vi "DispenseOnly.vi"() -> ()   [LabVIEW 2019]
uses:
  Other Models/EFD Ultimus V/EFD Ultimus V.lvlib
panel:
  in  "ActualDispense":bool
  out "NewPatternPressure":dbl[](array[numeric])
  out "AmtDispensed(g)":dbl
  out "CorrectionFactor":dbl=1.0
  in  "WtFor50Psi30Sec":dbl=1.039
  in  "PaperWtWithGlue(g)":dbl
  in  "PaperWt(g)":dbl
  in  "PatternPressDefault":dbl[](array[numeric])=[30.0, 21.0, 0.0, 0.0]
  out "TimeCalculated":dbl
  out "error out":errorcluster
  in  "Serial Configuration":T1={"Baud Rate "=115200, "Parity "=0, "Data Bits "=8, "Stop Bits"=10} {"Stop Bits" items=["1.0"=10, "1.5"=15, "2.0"=20]; "Data Bits" items=["7"=7, "8"=8]; "Parity" items=["None", "Odd", "Even"]; "Baud Rate" items=["9600"=9600, "19200"=19200, "38400"=38400, "115200"=115200]}
  in  "VISA resource name":refnum<visa-resource-name>="COM5"
  in  "Time(s)":dbl=30.0
  in  "PressureSet":dbl=50.0
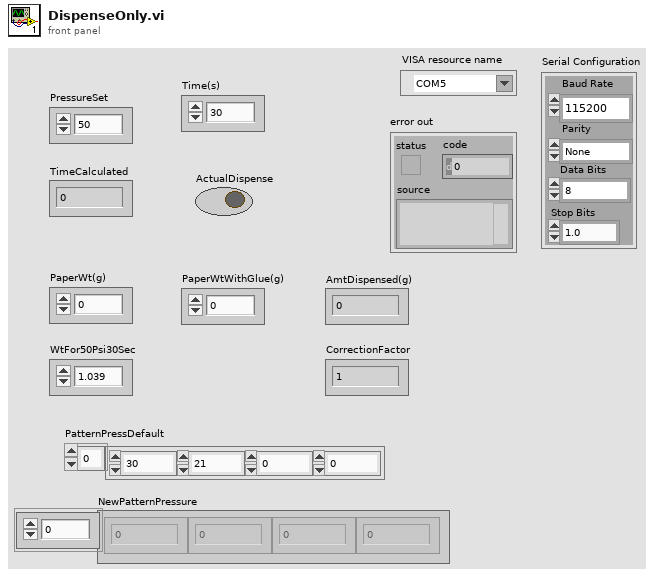
[diagram p1: front panel]
types:
  T1 = cluster{"Baud Rate ":u32, "Parity ":u16, "Data Bits ":u16, "Stop Bits":u16}
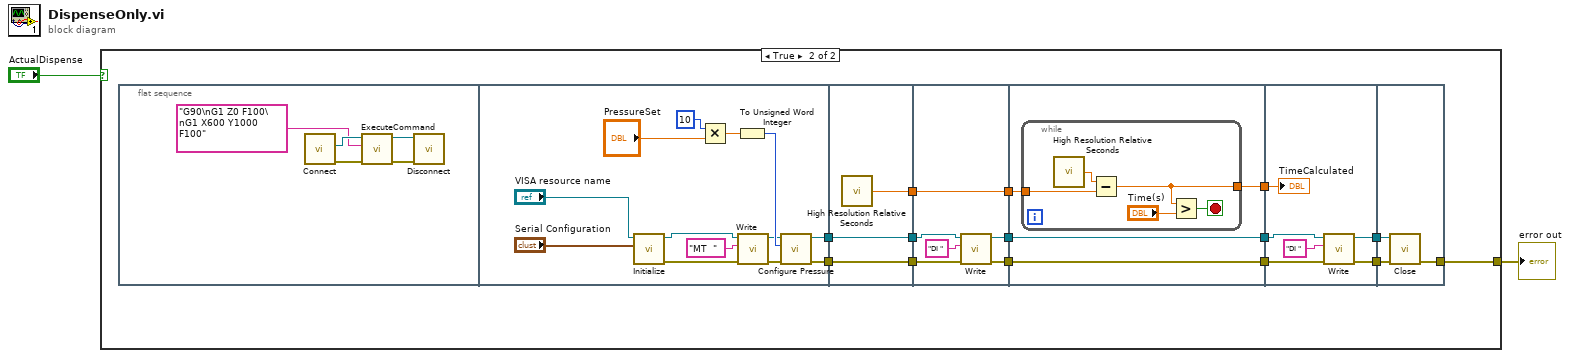
[diagram p0: block diagram]
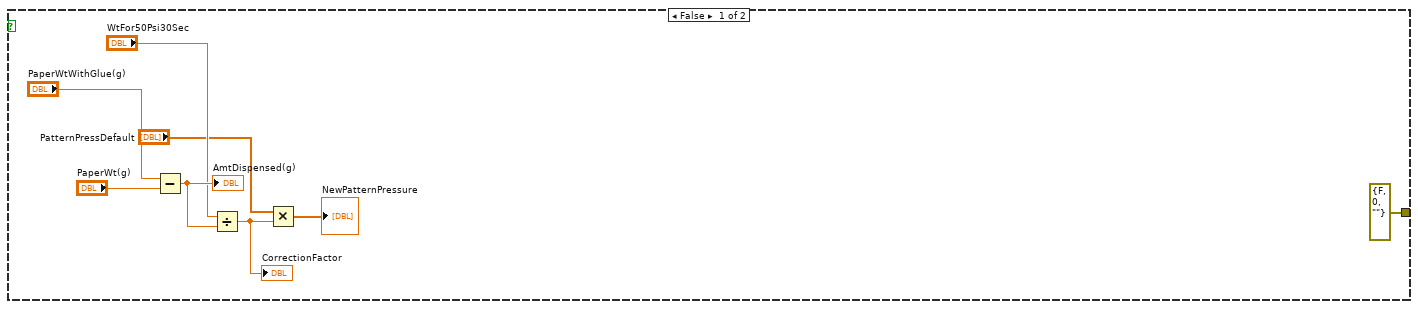
[diagram p2: hidden frame]
diagram:
  n1 = case shown="True" "ActualDispense" {
    tunnel: [errorcluster {"status"=FALSE, "code"=0, "source"=""} ("error in (no error)") w11] -> w2
    frame False {
      n2 = Subtract(x="PaperWtWithGlue(g)", y="PaperWt(g)") -> (x-y=w8:dbl)
      "AmtDispensed(g)" <- w8
      n3 = Divide(x="WtFor50Psi30Sec", y=w8) -> (x/y=w5:dbl)
      "CorrectionFactor" <- w5
      n4 = Multiply(x="PatternPressDefault", y=w5) -> (x*y=→"NewPatternPressure":dbl[])
    }
    frame True {
      n5 = flat-sequence {
        tunnel: [w30] -> w24
        tunnel: [w31] -> w23
        tunnel: [w45] -> w22
        tunnel: [w44] -> w21
        tunnel: [w43] -> w20
        tunnel: w24 -> [w45]
        tunnel: w23 -> [w44]
        tunnel: [w49] -> w19
        tunnel: [w48] -> w18
        tunnel: w22 -> [w51]
        tunnel: w21 -> [w50]
        tunnel: [w46] -> w17
        tunnel: w20 -> [w46]
        tunnel: w19 -> [w55]
        tunnel: w18 -> [w54]
        tunnel: [w55] -> w16
        tunnel: [w54] -> w15
        tunnel: w17 -> [w53]
        tunnel: [w52] -> w14
        tunnel: w16 -> [w65]
        tunnel: w15 -> [w66]
        tunnel: w14 -> [w61]
        tunnel: [w64] -> w13
        tunnel: [w63] -> w12
        tunnel: w13 -> [w69]
        tunnel: w12 -> [w68]
        tunnel: [w67] -> w11
        frame #0 {
          n6 = call "Connect.vi"() -> ("error out"=w28:errorcluster, "controller"=w29:refnum<k24>)  [unwired: 10 in]
          n7 = call "ExecuteCommand.vi"("error in (no error)"=w28, "Command Code"="G90\nG1 Z0 F100\nG1 X600 Y1000 F100", "controller in"=w29) -> ("error out"=w26:errorcluster, "controller out"=w27:refnum<k24>)  [unwired: 6 in, 1 out]
          n8 = call "Disconnect.vi"("error in (no error)"=w26, "controller"=w27) -> ()  [unwired: 9 in, 1 out]
        }
        frame #1 {
          n9 = call "Initialize.vi"("Serial Configuration"="Serial Configuration", "VISA resource name"="VISA resource name") -> ("error out"=w37:errorcluster, "VISA resource name out"=w36:refnum<visa-resource-name>)  [unwired: 8 in]
          n10 = Multiply(x=10, y="PressureSet") -> (x*y=w39:dbl)
          n11 = To Unsigned Word Integer(number=w39) -> (unsigned 16bit integer=w40:u16)
          n12 = call "Write.vi"("error in (no error)"=w37, "Command To Write"="MT  ", "VISA resource name"=w36) -> ("error out"=w41:errorcluster, "VISA resource name out"=w38:refnum<visa-resource-name>)  [unwired: 7 in]
          n13 = call "Configure Pressure.vi"("error in (no error)"=w41, "Pressure Setting (0000)"=w40, "VISA resource name"=w38) -> ("error out"=w31:errorcluster, "VISA resource name out"=w30:refnum<visa-resource-name>)  [unwired: 7 in]
        }
        frame #2 {
          n14 = call <vilib>:"High Resolution Relative Seconds.vi"() -> ("relative seconds"=w43:dbl)
        }
        frame #3 {
          n15 = call "Write.vi"("error in (no error)"=w50, "Command To Write"="DI ", "VISA resource name"=w51) -> ("error out"=w48:errorcluster, "VISA resource name out"=w49:refnum<visa-resource-name>)  [unwired: 7 in]
        }
        frame #4 {
          n16 = while {
            tunnel: w53 -> [w59]
            tunnel: [w56] -> w52
            stop <- w58 stop-if-true
            n17 = call <vilib>:"High Resolution Relative Seconds.vi"() -> ("relative seconds"=w60:dbl)
            n18 = Subtract(x=w60, y=w59) -> (x-y=w56:dbl)
            n19 = Greater?(x=w56, y="Time(s)") -> (0:w58:bool)
          }
        }
        frame #5 {
          n20 = call "Write.vi"("error in (no error)"=w66, "Command To Write"="DI ", "VISA resource name"=w65) -> ("error out"=w64:errorcluster, "VISA resource name out"=w63:refnum<visa-resource-name>)  [unwired: 7 in]
          "TimeCalculated" <- w61
        }
        frame #6 {
          n21 = call "Close.vi"("error in (no error)"=w69, "VISA resource name"=w68) -> ("error out"=w67:errorcluster)  [unwired: 9 in]
        }
      }
    }
  }
  "error out" <- w2
